vi "testTypecast.vi"() -> ()   [LabVIEW 2009]
uses:
  shared programs/PolyRead/BooleanRead.vi
  shared programs/PolyWrite/TCP connection.vi
  shared programs/PolyWrite/DBL.vi
  shared programs/PolyWrite/Boolean.vi
panel:
  out "value":bool
  out "error out":errorcluster={"status"=FALSE, "code"=556, "source"=""}
  out "array out":string[][](array[string])
  in  "Boolean 2":bool=TRUE
  out "data 2":i32
  out "Array":string[](array[string])
  out "data":errorcluster
  out "data string":string
  in  "reference":refnum<vi>
  in  "generic class reference 2":refnum<vi>
  out "Class Name 2":string
  out "Array Reference":refnum<vi>
  in  "error":errorcluster
  in  "Path":path
  in  "connection ID":refnum<k16>
  in  "DBl":dbl format="%#_6e"
  in  "Boolean":bool=TRUE
  in  "I32":i32
  in  "string":string="init: read config file"
  in  "Array in":string[](array[string])
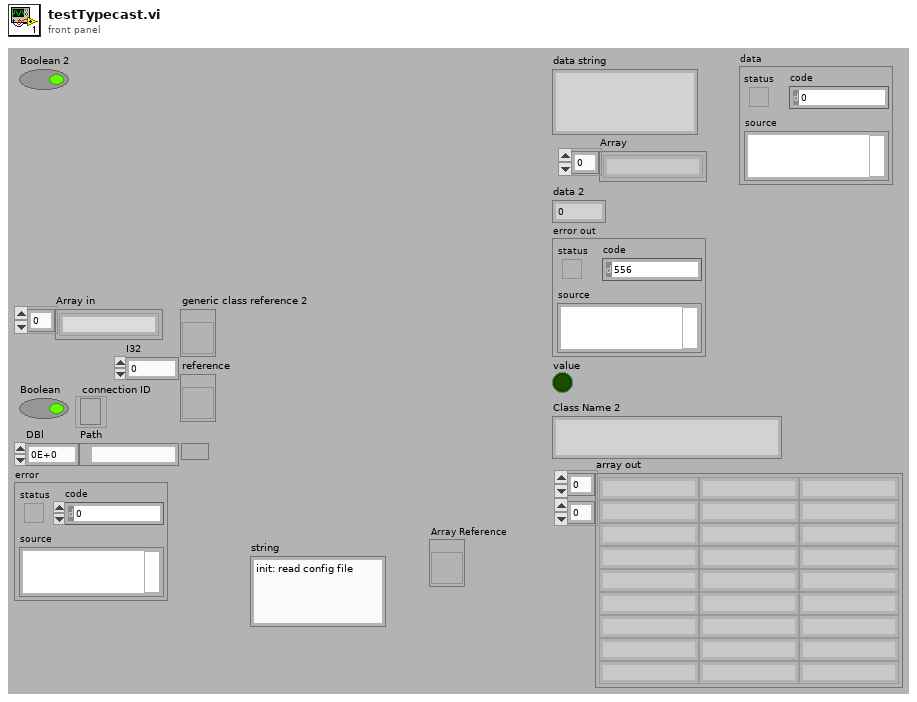
[diagram p1: front panel]
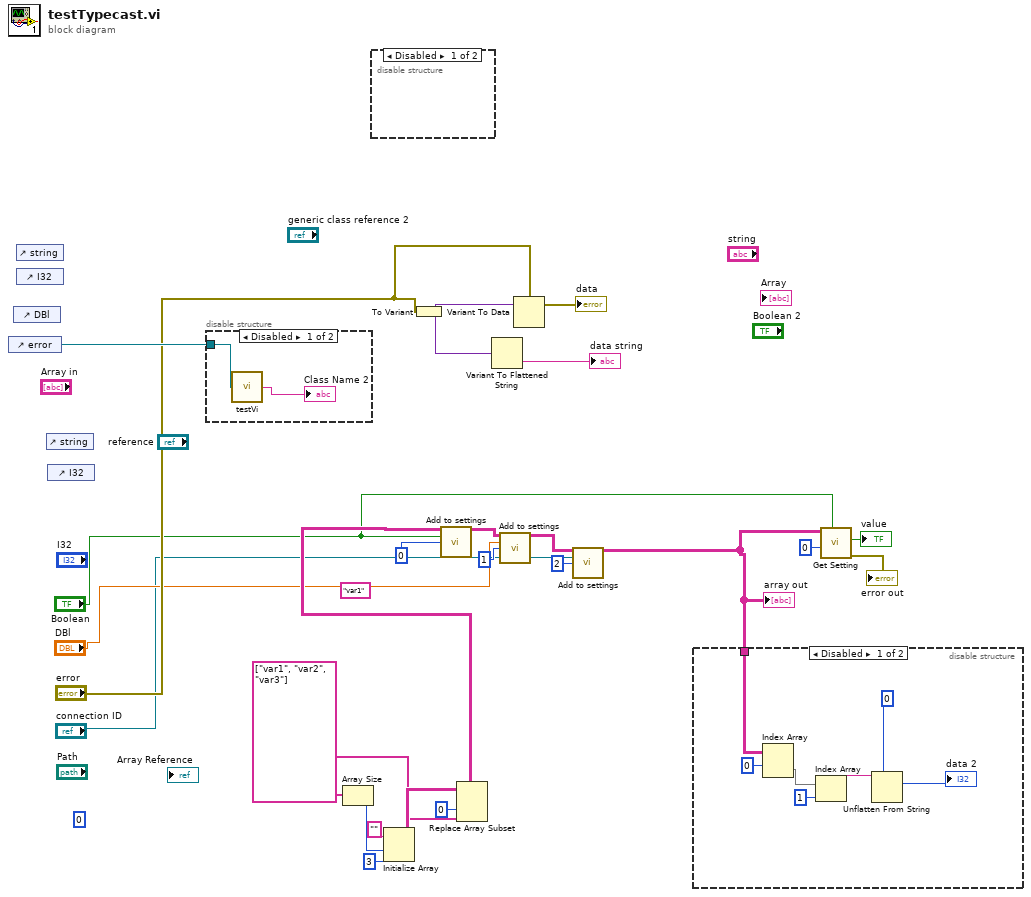
[diagram p0: block diagram]
diagram:
  w14 = string[] ["var1", "var2", "var3"]
  (unwired) "var1"
  (unwired) 0
  n1 = control-ref of="error"() -> (w24:refnum<vi>)
  n2 = control-ref of="DBl"() -> ()  [unwired: 1 out]
  n3 = control-ref of="string"() -> ()  [unwired: 1 out]
  n4 = control-ref of="I32"() -> ()  [unwired: 1 out]
  n5 = control-ref of="string"() -> ()  [unwired: 1 out]
  n6 = control-ref of="I32"() -> ()  [unwired: 1 out]
  n7 = disable-structure shown="Disabled" {
    disable-tunnel: w24 -> [w25 _]
    frame #0 {
      n8 = call "testVi.vi"("reference"=w25) -> ("Class Name 2"=→"Class Name 2":string)
    }
    frame #1 {
    }
  }
  n9 = Array Size(array=w14) -> (size(s)=w17:i32)
  n10 = disable-structure shown="Disabled" {
    frame #0 {
    }
    frame #1 {
    }
  }
  n11 = Initialize Array("" ("string"), w17, 3 ("dimension size")) -> (w16:string[][])
  n12 = To Variant(anything="error") -> (Variant=w22:variant)
  n13 = Replace Array Subset(array=w16, new element=w14, index (col)=0 ("disabled index (col)")) -> (w13:string[][])  [unwired: 1 in]
  n14 = call-poly "Add to settings.vi"("array in"=w13, "Boolean"="Boolean", "index"=0 ("I32")) -> ("array out"=w11:string[][])  [unwired: 11 in, 1 out]
  n15 = Variant To Flattened String(Variant=w22) -> (data string=→"data string":string)  [unwired: 1 out]
  n16 = call-poly "Add to settings.vi"("array in"=w11, "DBl"="DBl", "index"=1) -> ("array out"=w8:string[][])  [unwired: 11 in, 1 out]
  n17 = Variant To Data(Variant=w22, type="error") -> (data=→"data":errorcluster)  [unwired: 1 in, 1 out]
  n18 = call-poly "Add to settings.vi"("array in"=w8, "connection ID"="connection ID", "index"=2) -> ("array out"=w6:string[][])  [unwired: 11 in, 1 out]
  "array out" <- w6
  n19 = disable-structure shown="Disabled" {
    disable-tunnel: w6 -> [w27 _]
    frame #0 {
      n20 = Index Array(array=w27, index (row)=0) -> (element=w32:string[])  [unwired: 1 in]
      n21 = Index Array(array=w32, index=1) -> (element=w30:string)
      n22 = Unflatten From String(type=0, binary string=w30) -> (value=→"data 2":i32)  [unwired: 3 in, 2 out]
    }
    frame #1 {
    }
  }
  n23 = call-poly "Get Setting.vi"("Boolean"="Boolean", "index"=0, "array in"=w6) -> ("error out"=→"error out":errorcluster, "value"=→"value":bool)  [unwired: 6 in, 1 out]
